vi "CS_Start.vi"() -> ()   [LabVIEW 2014]
doc: "\"Main\" of a CS system on the local machine. Mailny the SuperProc should be started from here. Other objects are created by the SuperProc itself. A list of names of all the objects to be created by the user is part of the data base (SuperProc->Special0-SpecialN).\n\nLicense Agreement for this software:\n\nCopyright (C) 2013 Holger Brand, Dennis Neidherr\nGSI Helmholtzzentrum für Schwerionenforschung GmbH\nPlanckstraße 1\nD-64291 Darmstadt\nGermany\n\nContact: d.neidherr@gsi.de \n\nThis program is free software: you can redistribute it and/or modify it under the terms\nof the GNU General Public License as published by the Free Software Foundation, either\nversion 3 of the License, or (at your option) any later version.\n\nThis program is distributed in the hope that it will be useful, but WITHOUT ANY WARRANTY;\nwithout even the implied warranty of MERCHANTABILITY or FITNESS FOR A PARTICULAR PURPOSE.\nSee the GNU General Public License for more details.\n\nYou should have received a copy of the GNU General Public License along with this program.\nIf not, see <http://www.gnu.org/licenses/>.\n\nFor all questions and ideas contact: d.neidherr@gsi.de or h.brand@gsi.de\nLast update: 20-Mar-2013\n\nmenuHelpStart\nFile\n==\n- \"Shutdown\" gently exits the CS system by removing all objects\n- \"Exit\" unfriendly exits the CS system by exiting the application without removing of objects. \n\nTools\n===\n- \"UserGOG\" displays a generic object GUI (GOG) for on-line testing purposes by the user sitting in front of the computer. If you would like to routinely open a GOG when a CS system starts, please configure a dedicated GOG via the database and configure the SuperProc to create that GOG upon starting up the system.\n\n- \"Inspector\" shows information on the objects of THIS and other CS systems.\n\n- \"DIM Table\" provides a simple possibility for viewing DIM services.\n\n- \"DIM Trend\" can be used for trending of DIM services\n\n- \"DIM Histogram\" can be used for histogramming of multiple DIM services\n\n- \"Access Viewer\" can be used to view the hierarchy of reserved objects. Moreover, it allows for locking the access to certain objects and sub-systems.\n\n- \"DSC Alarm Viewer\" is the alarm viewer of the SCADA backend based on the LabVIEW DSC module. When using the alarm viewer, you will be asked for the name of the DSC interface. The alarm viewer requires a binary compiled with the CSDSC_SCADA package.\nmenuHelpStop\n\ndescriptionHelpStart\n\"Main\" of a CS instance. CS is a framework that can be used by many experiments. CS is a multi-threaded, event driven, object oriented and distributed framework with SCADA functionality. An experiment control system can be developed by combining the CS framework with experiment specific add-ons.\n\nMore information available at http://wiki.gsi.de/cgi-bin/view/CSframework\n\ndescriptionHelpStop"
uses:
  CSClass/CS_Core/GUIs/GOGFrontPanel/GOGFrontPanel.i attribute.ctl
  CSClass/CS_Core/BaseProcess/BaseProcess.descriptor string definition.ctl
  CSClass/CS_Core/CSSystem/CSSystemLib/CSSystemLib.instances options.ctl
  CSlibraries-extern/DimLVEvent/LVDimInterface/LVDimInterface.dim service type.ctl
  CSlibraries/UtilityLib/UtilityLib.helpType.ctl
  CSClass/CS_Core/CSSystem/CoreDefs/CoreDefs.error_severity.ctl
  CSClass/CS_Core/CSSystem/CoreDefs/CoreDefs.error_type.ctl
  CSlibraries/UtilityLib/UtilityLib.valueStatus.ctl
  CSlibraries-extern/DimLVEvent/LVDimInterface/LVDimInterface.dic_info_service_notifier.vi
  CSClass/CS_Core/CSSystem/CoreLib/CoreLib.lvlib
  CSlibraries-extern/DimLVEvent/LVDimInterface/LVDimInterface.lvlib
  CSClass/CS_Core/CSSystem/CSSystemLib/CSSystemLib.lvlib
  CSClass/CS_Core/BaseProcess/BaseProcess.lvlib
  CSlibraries/UtilityLib/UtilityLib.lvlib
  CSClass/CS_Core/CSObj/CSObj.lvlib
  CSClass/CS_Core/CAEObj/CAEObj.lvlib
  CSClass/CS_Core/BaseSM/BaseSM.lvlib
  CSClass/CS_Core/BaseGUI/BaseGUI.lvlib
  CSClass/CS_Core/GUIs/GOGFrontPanel/GOGFrontPanel.lvlib
panel:
  in  "False":bool
  out "database":string="Process@"
  out "domainInfo":string="hello world :-)"
  in  "GOGFrontPanel.i attribute":T1
  out "system running":bool=TRUE
  out "status":string="shutting down..."
  out "systemID":string="TestSystem@KSTest@lxgs11.gsi.de"
  out "error out":errorcluster
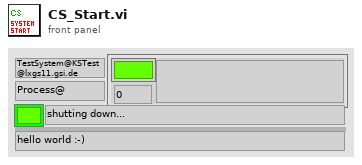
[diagram p1: front panel]
types:
  T1 = typedef "GOGFrontPanel.lvlib/GOGFrontPanel.i attribute.ctl" = cluster{"GOGObject":string, "Object":string, "Method":string, "Descriptor":T2, "Input Descriptor":string, "Output Descriptor":string, "inputNames":string[], "outputNames":string[], "Values":cluster{"descriptor":string, "value":string}[]}
  T2 = typedef "BaseProcess.lvlib/BaseProcess.descriptor string definition.ctl" = string
  T3 = enum32{"Invalid", "Standard", "Closed", "Hidden", "Minimized", "Maximized"}
  T4 = enum32{"invalid app kind", "Development System", "Run Time System", "Student Edition", "Embedded LabVIEW", "Evaluation", "Custom"}
  T5 = typedef "CSSystemLib.lvlib/CSSystemLib.instances options.ctl" = enum16{"add", "delete", "name2ref", "ref2name ", "ref2class", "obj exists?", "cleanup", "get I list", "get I list all", "ref2myclasses", "setClassNames"}
  T6 = enum16{"acquire queue", "release queue", "destroy queue", "get command ID", "destroy all queues"}
  T7 = typedef "UtilityLib.lvlib/UtilityLib.helpType.ctl" = enum16{"unknown", "menu", "description", "about", "special0", "special1", "special2"}
  T8 = typedef "CoreDefs.error_type.ctl" = enum16{"no error", "can't load process", "can't unload process", "process does not exist", "can't install process", "can't remove process", "unknown function", "time out", "can't execute function", "duplicate queue name", "super not found", "caller queue invalid", "can't ping process", "unknown error", "VISA Error", "VISA timeout", "GPIB timeout", "GPIB error", "communication error", "data type mismatch", "can't read data from OPC server", "can't write data to OPC server", "OET error", "function not implemented", "process already exists", "invalid Shared Variable name", "error writing Shared Variable", "error reading Shared Variable", "invalid client name", "corrupt database", "unknown class", "call not authorized", "parameter out of range", "OET timeout: can't get data to modify", "invalid queue name", "requested operation incompatible with current state", "event undefined", "event disabled", "state undefined", "caller is not a friend", "EventBuilder: bad eventID", "EventBuilder: no DAQ devices", "a thread must not stop itself", "UNUSED ELEMENT4", "DiscArchiver: eventData incomplete", "DiscArchiver: eventData does not belong to run", "DiscArchiver: can't open file", "DiscArchiver: can't write to file", "DiscArchiver: available disc space low", "can't acquire semaphore", "error reading data from database", "notifier object is not existing", "can't register process", "can't unregister process", "illegal event type", "object disabled", "object already exists", "can't change state", "Instrument not found", "no connection to remote node", "invalid reference", "N/A", "UNUSED ELEMENT 1", "element not found", "illegal TCP/IP connection detected", "object does not exist", "invalid access ID", "unknown CS system", "invalid privilige", "unsupported data type", "unsupported server type", "IO server already exists", "Shared Variable already exists"}
  T9 = typedef "CoreDefs.error_severity.ctl" = enum16{"undefined", "information", "warning", "error", "fatal"}
  T10 = typedef "UtilityLib.lvlib/UtilityLib.valueStatus.ctl" = enum16{"no info available", "stand by/off", "on", "warning", "alarm/malfunction", "not implemented", "user action required", "important information", "system default", "control default", "indicator default", "button default"}
  T11 = enum32{"Bad", "Idle", "Run top level", "Running"}
  T12 = typedef "LVDimInterface.lvlib/LVDimInterface.dim service type.ctl" = u16
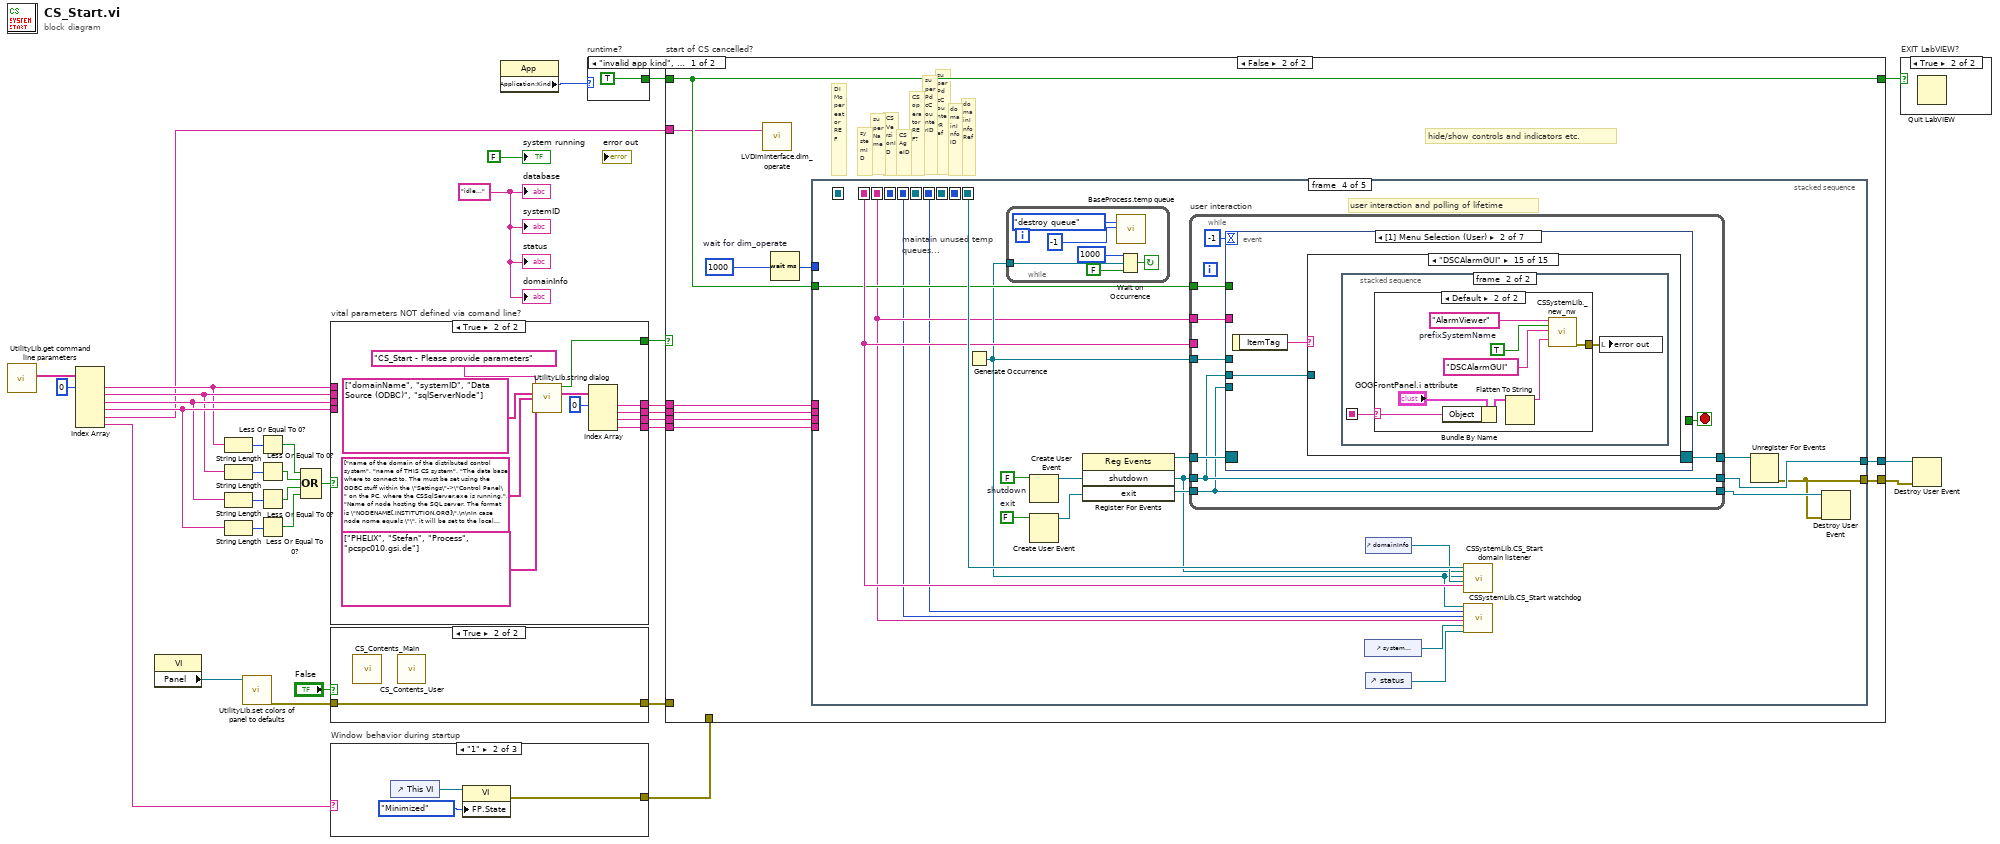
[diagram p0: block diagram]
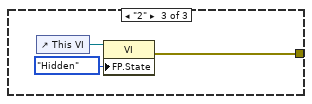
[diagram p3: hidden frame]
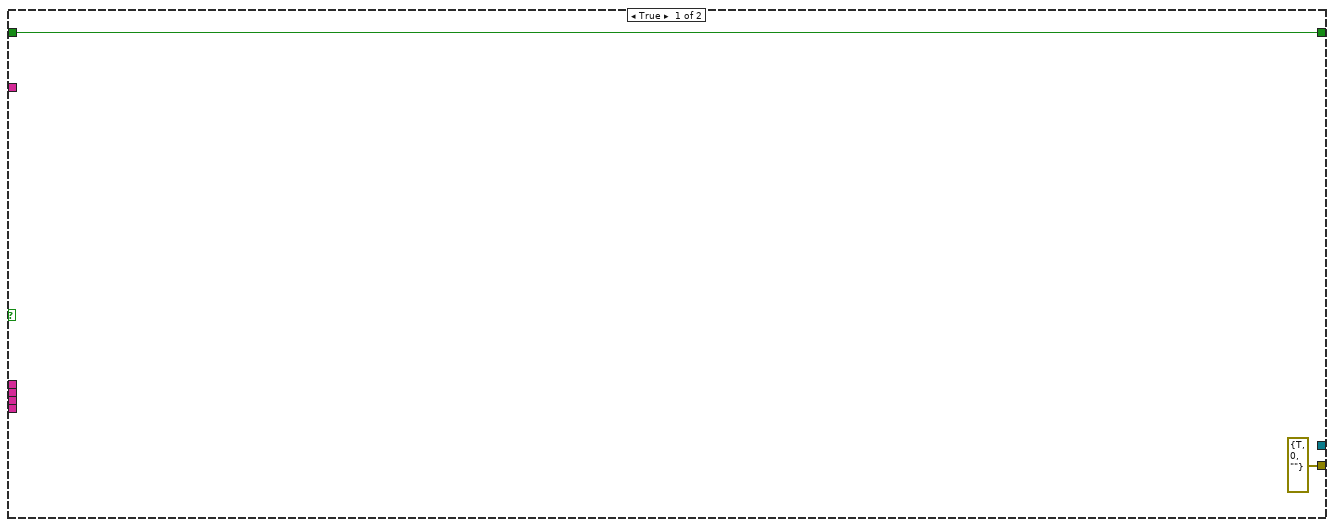
[diagram p6: hidden frame]
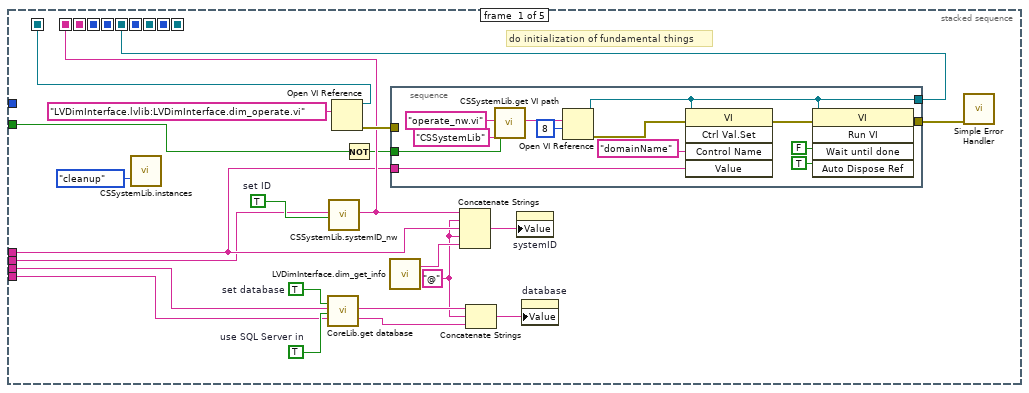
[diagram p7: hidden frame]
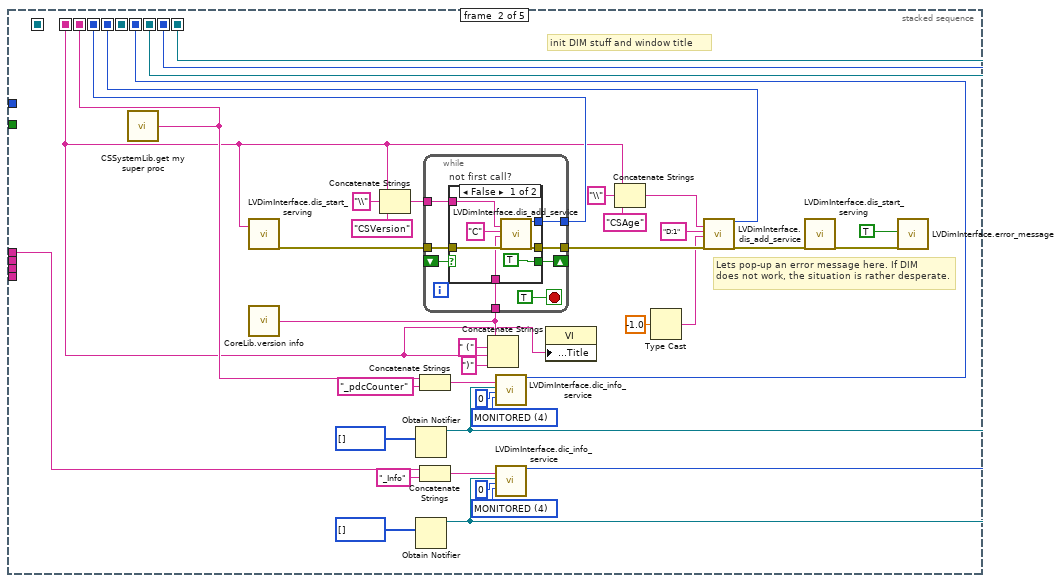
[diagram p8: hidden frame]
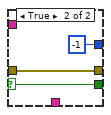
[diagram p9: hidden frame]
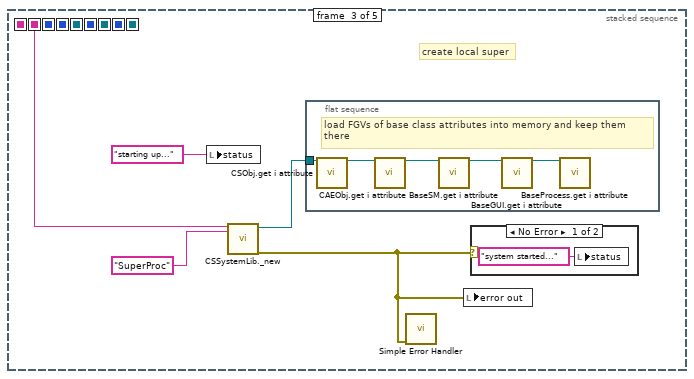
[diagram p10: hidden frame]
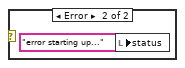
[diagram p11: hidden frame]
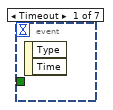
[diagram p12: hidden frame]
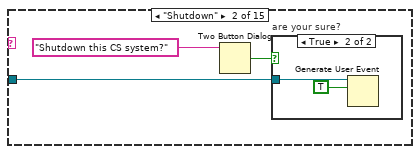
[diagram p14: hidden frame]
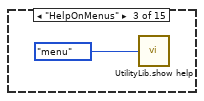
[diagram p16: hidden frame]
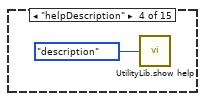
[diagram p17: hidden frame]
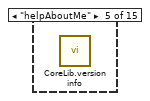
[diagram p18: hidden frame]
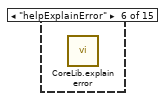
[diagram p19: hidden frame]
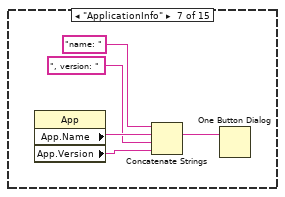
[diagram p20: hidden frame]
diagram:
  w13 = "idle..." ("status")
  n1 = call "UtilityLib.get command line parameters.vi"() -> ("parametersCleaned"=w3:string[])  [unwired: 9 in, 2 out]
  n2 = Index Array(array=w3, index #1=0 ("index")) -> (element #1=w21:string, element #2=w23:string, element #3=w25:string, element #4=w32:string, element #5=w8:string, element #6=w5:string)  [unwired: 5 in]
  n3 = property class="VI"() -> ("Panel"=w9:refnum<vi>)  [unwired: 2 in, 2 out]
  n4 = String Length(string=w21) -> (length=w20:i32)
  n5 = String Length(string=w23) -> (length=w22:i32)
  n6 = String Length(string=w25) -> (length=w24:i32)
  n7 = String Length(string=w32) -> (length=w30:i32)
  n8 = call "UtilityLib.set colors of panel to defaults.vi"("Front Panel"=w9) -> ("error out"=w12:errorcluster)  [unwired: 18 in]
  n9 = Less Or Equal To 0?(x=w20) -> (x <= 0?=w26:bool)
  n10 = Less Or Equal To 0?(x=w22) -> (x <= 0?=w27:bool)
  n11 = Less Or Equal To 0?(x=w24) -> (x <= 0?=w28:bool)
  n12 = Less Or Equal To 0?(x=w30) -> (x <= 0?=w31:bool)
  n13 = Compound Arithmetic op=OR(w26, w27, w28, w31) -> (w29:bool)
  n14 = case "vital parameters NOT defined via comand line?" shown="True" w29 {
    tunnel: [w38 w44] -> w17
    tunnel: w21 -> [w38 _]
    tunnel: [w37 w42] -> w2
    tunnel: w23 -> [w37 _]
    tunnel: w25 -> [w36 _]
    tunnel: [w36 w43] -> w16
    tunnel: w32 -> [w35 _]
    tunnel: [w35 w40] -> w15
    tunnel: [_ w41] -> w6
    frame False {
    }
    frame True {
      n15 = call "UtilityLib.string dialog.vi"("title"="CS_Start - Please provide parameters", "captions"=string[] ["domainName", "systemID", "Data Source (ODBC)", "sqlServerNode"], "helpText"=string[] ["name of the domain of the distributed control system", "name of THIS CS system", "The data base where to connect to. The must be set using the ODBC stuff within the \"Settings\"->\"Control Panel\" on the PC, where the CSSqlServer.exe is running.", "Name of node hosting the SQL server. The format is \"NODENAME[.INSTITUTION.ORG]\".\n\nIn case node nome equals \"\", it will be set to the local host."], "initialValue"=string[] ["PHELIX", "Stefan", "Process", "pcspc010.gsi.de"]) -> ("cancelled"=w41:bool, "strings"=w46:string[])  [unwired: 8 in, 2 out]
      n16 = Index Array(array=w46, index #1=0 ("index")) -> (element #1=w44:string, element #2=w42:string, element #3=w43:string, element #4=w40:string)  [unwired: 3 in]
    }
  }
  n17 = case shown="True" "False" {
    tunnel: w12 -> [w50 w51]
    tunnel: [w50 w51] -> w11
    frame False {
    }
    frame True {
      n18 = call "CS_Contents_Main.vi"() -> ()  [unwired: 1 in]
      n19 = call "CS_Contents_User.vi"() -> ()  [unwired: 1 in]
    }
  }
  n20 = case "Window behavior during startup" shown="\"1\"" w5 {
    tunnel: [_ w54 w55] -> w7
    frame Default {
    }
    frame "1" {
      n21 = control-ref of="This VI"() -> (w52:refnum<vi>)
      n22 = property class="VI"(reference=w52, "FP.State"=T3."Minimized" ("Front Panel Window:State")) -> (error out=w54:errorcluster)  [unwired: 1 in, 1 out]
    }
    frame "2" {
      n23 = control-ref of="This VI"() -> (w57:refnum<vi>)
      n24 = property class="VI"(reference=w57, "FP.State"=T3."Hidden" ("Front Panel Window:State")) -> (error out=w55:errorcluster)  [unwired: 1 in, 1 out]
    }
  }
  n25 = property class="App"() -> ("Application:Kind"=w34:T4)  [unwired: 2 in, 2 out]
  n26 = case "runtime?" shown="\"invalid app kind\", Default" w34 {
    tunnel: [TRUE _] -> w19
    frame "invalid app kind", Default {
    }
    frame "Development System" {
    }
  }
  n27 = case "start of CS cancelled?" shown="False" w6 {
    tunnel: w19 -> [w60 w70]
    tunnel: [w60 w70] -> w18
    tunnel: w8 -> [_ w69]
    tunnel: w17 -> [_ w68]
    tunnel: w2 -> [_ w61]
    tunnel: w16 -> [_ w67]
    tunnel: w15 -> [_ w66]
    tunnel: w11 -> [_ _]
    tunnel: w7 -> [_ _]
    tunnel: [_ w63] -> w4
    tunnel: [errorcluster {"status"=TRUE, "code"=0, "source"=""} ("error out") w62] -> w1
    frame True {
    }
    frame False {
      # "hide/show controls and indicators etc."
      # "domainInfoRef"
      # "domainInfoID"
      # "superPdcCounterRef"
      # "superPdcCounterID"
      # "CSoperator REF?"
      # "CSAgeID"
      # "CSVersionID"
      # "superName"
      # "systemID"
      # "DIMopereator REF"
      n28 = call "LVDimInterface.dim_operate.vi"("DNSNode"=w69) -> ()  [unwired: 19 in]
      n29 = Wait (ms) "wait for dim_operate"(milliseconds to wait=u32 1000) -> (millisecond timer value=w64:u32)
      n30 = stacked-sequence {
        seq-local: [w83 _ _ _ _] -> [_ w106 _ w189 _]
        seq-local: [w90 _ _ _ _] -> [_ _ _ _ w304]
        seq-local: [_ w115 _ _ _] -> [_ _ w162 w182 _]
        seq-local: [_ w130 _ _ _] -> [_ _ _ _ w300]
        seq-local: [_ w129 _ _ _] -> [_ _ _ w178 w299]
        seq-local: [w91 _ _ _ _] -> [_ _ _ _ w303]
        seq-local: [_ w119 _ _ _] -> [_ _ _ w179 w297]
        seq-local: [_ w118 _ _ _] -> [_ _ _ _ w295]
        seq-local: [_ w109 _ _ _] -> [_ _ _ _ w289]
        seq-local: [_ w108 _ _ _] -> [_ _ _ w190 w288]
        tunnel: w70 -> [w73 _ _ w185 w287]
        tunnel: w68 -> [w82 w107 _ _ _]
        tunnel: w61 -> [w71 _ _ _ _]
        tunnel: w67 -> [w86 _ _ _ _]
        tunnel: w66 -> [w85 _ _ _ _]
        tunnel: w64 -> [_ _ _ _ _]
        tunnel: [_ _ _ w177 _] -> w63
        tunnel: [_ _ _ w176 _] -> w62
        frame #0 {
          w80 = "@" ("string")
          w89 = TRUE  # use SQL Server in
          w92 = TRUE  # set database
          w72 = TRUE  # set ID
          # "do initialization of fundamental things"
          n31 = call "CSSystemLib.instances.vi"("Action"=CSSystemLib.instances_options."cleanup") -> ()  [unwired: 12 in, 7 out]
          n32 = call "CoreLib.get database.vi"("set database"=w92, "database in"=w86, "use SQL Server in"=w89, "SQL Server node in"=w85) -> ("database"=w81:string, "SQL Server node"=w79:string)  [unwired: 12 in, 2 out]
          n33 = call "CSSystemLib.systemID_nw.vi"("systemID"=w71, "Force set ID"=w72) -> ("systemID out"=w83:string)  [unwired: 16 in, 1 out]
          n34 = Open VI Reference(vi path="LVDimInterface.lvlib:LVDimInterface.dim_operate.vi") -> (vi reference=w90:refnum<vi>, error out=w87:errorcluster)  [unwired: 5 in]
          n35 = Not(x=w73) -> (.not. x?=w74:bool)
          n36 = call "LVDimInterface.dim_get_info.vi"() -> ("dimDnsNode"=w84:string)  [unwired: 13 in, 6 out]
          n37 = stacked-sequence {
            tunnel: w82 -> [w97]
            tunnel: [w101] -> w91
            tunnel: [w100] -> w75
            tunnel: w87 -> [_]
            tunnel: w74 -> [w94]
            frame #0 {
              n38 = call "CSSystemLib.get VI path.vi"("method"="operate_nw.vi" ("Method"), "class"="CSSystemLib" ("Class"), "reReead"=w94) -> ("VI path"=w96:string)  [unwired: 14 in, 2 out]
              n39 = Open VI Reference(vi path=w96, options=8) -> (vi reference=w101:refnum<vi>, error out=w104:errorcluster)  [unwired: 4 in]
              n40 = invoke class="VI" method="Ctrl Val.Set"(reference=w101, error in=w104, "Control Name"="domainName", "Value"=w97) -> (error out=w103:errorcluster)  [unwired: 1 in, 4 out]
              n41 = invoke class="VI" method="Run VI"(reference=w101, error in=w103, "Wait until done"=FALSE, "Auto Dispose Ref"=TRUE ("Auto Dispose Reference")) -> (error out=w100:errorcluster)  [unwired: 1 in, 4 out]
            }
          }
          n42 = Concatenate Strings(w83, w80, w82, w80, w84) -> (w78:string)
          n43 = Concatenate Strings(w81, w80, w79) -> (w77:string)
          n44 = property on="systemID" class="Str"("Value"=w78) -> ()  [unwired: 2 in, 2 out]
          n45 = property on="database" class="Str"("Value"=w77) -> ()  [unwired: 2 in, 2 out]
          n46 = call <vilib>:"Simple Error Handler.vi"("error in (no error)"=w75) -> ()  [unwired: 4 in, 5 out]
        }
        frame #1 {
          w114 = T12 4 items=["ONCE_ONLY"=1, "TIMED"=2, "MONITORED"=4] ("serviceType")
          w116 = T12 4 items=["ONCE_ONLY"=1, "TIMED"=2, "MONITORED"=4] ("serviceType")
          # "Lets pop-up an error message here. If DIM\ndoes not work, the situation is rather desperate."
          # "init DIM stuff and window title"
          n47 = call "CSSystemLib.get my super proc.vi"() -> ("name"=w115:string)  [unwired: 1 in]
          n48 = call "LVDimInterface.dis_start_serving.vi"("serverName"=w106) -> ("error out"=w138:errorcluster)  [unwired: 17 in, 1 out]
          n49 = call "CoreLib.version info.vi"() -> ("CS Version"=w126:string)  [unwired: 4 in, 1 out]
          n50 = Concatenate Strings(w106, "\\" ("string"), "CSVersion" ("string")) -> (w141:string)
          n51 = Obtain Notifier(notification data type=i8[] []) -> (notifier out=w118:refnum<notifier>)  [unwired: 3 in, 2 out]
          n52 = Obtain Notifier(notification data type=i8[] []) -> (notifier out=w108:refnum<notifier>)  [unwired: 3 in, 2 out]
          n53 = Concatenate Strings(w115, "_pdcCounter" ("string")) -> (w121:string)
          n54 = Concatenate Strings(w107, "_Info" ("string")) -> (w111:string)
          n55 = while {
            tunnel: w141 -> [w149]
            tunnel: w138 -> [w148]
            tunnel: [w147] -> w134
            tunnel: [w146] -> w130
            tunnel: w126 -> [w145]
            shift-right: [w143] -> _
            shift-left: _ -> [w142]
            stop <- TRUE stop-if-true
            n56 = case "not first call?" shown="False" w142 {
              selector: w142 -> [_ w157]
              tunnel: w149 -> [w156 _]
              tunnel: w148 -> [w154 w159]
              tunnel: [w153 w159] -> w147
              tunnel: [w152 -1 ("my_serviceID")] -> w146
              tunnel: w145 -> [w151 _]
              tunnel: [TRUE w157] -> w143
              frame False {
                n57 = call "LVDimInterface.dis_add_service.vi"("serviceName"=w156, "typeDescriptor"="C", "data"=w151, "error in (no error)"=w154) -> ("my_serviceID"=w152:i32, "error out"=w153:errorcluster)  [unwired: 14 in]
              }
              frame True {
              }
            }
          }
          n58 = Concatenate Strings(w126, " (" ("string"), w106, ")" ("string")) -> ()  [unwired: 1 out]
          n59 = call-poly "LVDimInterface.dic_info_service.vi"("serviceName"=w121, "notifierRef"=w118, "timeout [s]"=0, "serviceType"=w116) -> ("callBackID"=w119:i32)  [unwired: 14 in, 1 out]
          n60 = call-poly "LVDimInterface.dic_info_service.vi"("serviceName"=w111, "notifierRef"=w108, "timeout [s]"=0, "serviceType"=w114) -> ("callBackID"=w109:i32)  [unwired: 14 in, 1 out]
          n61 = property class="VI"("Front Panel Window:Title"=w106) -> ()  [unwired: 2 in, 2 out]
          n62 = Concatenate Strings(w106, "\\" ("string"), "CSAge" ("string")) -> (w137:string)
          n63 = Type Cast(x=-1.0) -> (*(type *) &x=w132:string)  [unwired: 1 in]
          n64 = call "LVDimInterface.dis_add_service.vi"("serviceName"=w137, "typeDescriptor"="D:1", "data"=w132, "error in (no error)"=w134) -> ("my_serviceID"=w129:i32, "error out"=w124:errorcluster)  [unwired: 14 in]
          n65 = call "LVDimInterface.dis_start_serving.vi"("error in (no error)"=w124) -> ("error out"=w123:errorcluster)  [unwired: 17 in, 1 out]
          n66 = call "LVDimInterface.error_message.vi"("add message to source"=TRUE, "error in (no error)"=w123) -> ()  [unwired: 14 in, 4 out]
        }
        frame #2 {
          # "create local super"
          n67 = local write "status"("starting up..." ("status")) -> ()
          n68 = call "CSSystemLib._new.vi"("object name"=w162, "class name"="SuperProc") -> ("i ref out"=w161:refnum<vi>, "error out"=w160:errorcluster)  [unwired: 14 in, 2 out]
          n69 = flat-sequence {
            tunnel: w161 -> [w169]
            frame #0 {
              # "load FGVs of base class attributes into memory and keep them\nthere"
              n70 = call "CSObj.get i attribute.vi"("i ref in"=w169) -> ("i ref out"=w168:refnum<vi>)  [unwired: 16 in, 2 out]
              n71 = call "CAEObj.get i attribute.vi"("i ref in"=w168) -> ("i ref out"=w167:refnum<vi>)  [unwired: 16 in, 2 out]
              n72 = call "BaseSM.get i attribute.vi"("i ref in"=w167) -> ("i ref out"=w166:refnum<vi>)  [unwired: 16 in, 2 out]
              n73 = call "BaseGUI.get i attribute.vi"("i ref in"=w166) -> ("i ref out"=w165:refnum<vi>)  [unwired: 16 in, 2 out]
              n74 = call "BaseProcess.get i attribute.vi"("i ref in"=w165) -> ()  [unwired: 16 in, 3 out]
            }
          }
          n75 = call <vilib>:"Simple Error Handler.vi"("error in (no error)"=w160) -> ()  [unwired: 4 in, 5 out]
          n76 = local write "error out"(w160) -> ()
          n77 = case shown="No Error" w160 {
            frame No Error {
              n78 = local write "status"("system started..." ("status")) -> ()
            }
            frame Error {
              n79 = local write "status"("error starting up..." ("status")) -> ()
            }
          }
        }
        frame #3 {
          w174 = FALSE  # exit
          w175 = FALSE  # shutdown
          # "user interaction and polling of lifetime"
          n80 = Generate Occurrence() -> (w183:refnum<k4>)
          n81 = while "maintain unused temp queues..." {
            tunnel: w183 -> [w194]
            stop <- w195 continue-if-true
            n82 = Wait on Occurrence(1:FALSE ("ignore previous (T)"), 2:w194, 3:1000 ("ms timeout (-1)")) -> (0:w195:bool)
            n83 = call "BaseProcess.temp queue.vi"("Action"=T6."destroy queue", "ID in"=-1) -> ()  [unwired: 14 in, 4 out]
          }
          n84 = Create User Event(user event datatype=w175) -> (user event=w172:refnum<user-event>)  [unwired: 1 in, 1 out]
          n85 = Create User Event(user event datatype=w174) -> (user event=w173:refnum<user-event>)  [unwired: 1 in, 1 out]
          n86 = register-events(w172, w173) -> (reference out=w188:refnum<event-registration>)  [unwired: 2 in, 1 out]
          n87 = while "user interaction" {
            tunnel: w183 -> [w205]
            tunnel: w182 -> [w203]
            tunnel: w189 -> [_]
            tunnel: w185 -> [w201]
            tunnel: w188 -> [w200]
            tunnel: w172 -> [w199]
            tunnel: [w198] -> w187
            tunnel: [w199] -> w177
            tunnel: w173 -> [w197]
            tunnel: [w197] -> w186
            stop <- w204 stop-if-true
            n88 = event shown="[1] Menu Selection (User)" {
              selector: w200 -> [_ _ _ _ _ _ _]
              dyn-events: [_ _ _ _ _ _ _] -> w198
              timeout: -1 -> [_ _ _ _ _ _ _]
              tunnel: w205 -> [_ _ _ w270 _ _ _]
              tunnel: w203 -> [_ _ _ w269 _ _ _]
              tunnel: [_ _ _ w268 _ _ _] -> w204
              tunnel: w201 -> [_ _ _ _ _ _ w282]
              tunnel: w199 -> [_ w206 _ _ _ _ _]
              tunnel: w197 -> [_ _ _ _ w277 w281 _]
              event Timeout {
                n89 = event-data() -> ()  [unwired: 1 in, 2 out]
              }
              event Menu Selection (User) {
                n90 = event-data() -> ("ItemTag"=w207:string)  [unwired: 1 in]
                n91 = case shown="\"DSCAlarmGUI\"" w207 {
                  tunnel: w206 -> [_ w208 _ _ _ _ _ _ _ _ _ _ _ _ _]
                  frame Default {
                  }
                  frame "Shutdown" {
                    n92 = Two Button Dialog(message="Shutdown this CS system?") -> (T button?=w209:bool)  [unwired: 2 in]
                    n93 = case "are your sure?" shown="True" w209 {
                      tunnel: w208 -> [_ w211]
                      frame False {
                      }
                      frame True {
                        n94 = Generate User Event(user event=w211, event data cluster=TRUE ("event data")) -> ()  [unwired: 2 in, 2 out]
                      }
                    }
                  }
                  frame "HelpOnMenus" {
                    n95 = call "UtilityLib.show help.vi"("helpType"=UtilityLib.helpType."menu") -> ()
                  }
                  frame "helpDescription" {
                    n96 = call "UtilityLib.show help.vi"("helpType"=UtilityLib.helpType."description") -> ()
                  }
                  frame "helpAboutMe" {
                    n97 = call "CoreLib.version info.vi"() -> ()  [unwired: 4 in, 2 out]
                  }
                  frame "helpExplainError" {
                    n98 = call "CoreLib.explain error.vi"() -> ()  [unwired: 1 in]
                  }
                  frame "ApplicationInfo" {
                    n99 = property class="App"() -> ("App.Name"=w217:string, "App.Version"=w215:string)  [unwired: 2 in, 2 out]
                    n100 = Concatenate Strings("name: " ("string"), w217, ", version: " ("string"), w215) -> (w219:string)
                    n101 = One Button Dialog(message=w219) -> ()  [unwired: 1 in, 1 out]
                  }
                  frame "UserGOG" {
                    w223 = TRUE  # prefixSystemName
                    n102 = call "CSSystemLib._new_nw.vi"("objectName"="UserGOG", "prefixSystemName"=w223, "className"="GeneralObjectGUI", "data in"="N/A") -> ("error out"=w222:errorcluster)  [unwired: 13 in, 2 out]
                    n103 = local write "error out"(w222) -> ()
                  }
                  frame "Inspector" {
                    w228 = TRUE  # prefixSystemName
                    n104 = call "CSSystemLib._new_nw.vi"("objectName"="Inspector" ("Data"), "prefixSystemName"=w228, "className"="ObjectInspector", "data in"="N/A") -> ("error out"=w227:errorcluster)  [unwired: 13 in, 2 out]
                    n105 = local write "error out"(w227) -> ()
                  }
                  frame "DIMTable" {
                    w233 = TRUE  # prefixSystemName
                    n106 = call "CSSystemLib._new_nw.vi"("objectName"="DIMTable" ("Data"), "prefixSystemName"=w233, "className"="DIMTableView", "data in"="N/A") -> ("error out"=w232:errorcluster)  [unwired: 13 in, 2 out]
                    n107 = local write "error out"(w232) -> ()
                  }
                  frame "DIMTrendGUI" {
                    w238 = TRUE  # prefixSystemName
                    n108 = call "CSSystemLib._new_nw.vi"("objectName"="DIMTrend" ("Data"), "prefixSystemName"=w238, "className"="DIMTrendGUI", "data in"="N/A") -> ("error out"=w237:errorcluster)  [unwired: 13 in, 2 out]
                    n109 = local write "error out"(w237) -> ()
                  }
                  frame "DIMHistogramGUI" {
                    w243 = TRUE  # prefixSystemName
                    n110 = call "CSSystemLib._new_nw.vi"("objectName"="DIMHistogram" ("Data"), "prefixSystemName"=w243, "className"="DIMHistogramGUI", "data in"="N/A") -> ("error out"=w242:errorcluster)  [unwired: 13 in, 2 out]
                    n111 = local write "error out"(w242) -> ()
                  }
                  frame "ToolsDispatchMessageBox" {
                    n112 = call "CSSystemLib.CS_Start dispatch message box.vi"() -> ("error out"=w245:errorcluster)  [unwired: 18 in, 1 out]
                    n113 = local write "error out"(w245) -> ()
                  }
                  frame "AccessViewer" {
                    w249 = TRUE  # prefixSystemName
                    n114 = call "CSSystemLib._new_nw.vi"("objectName"="AccessViewer" ("Data"), "prefixSystemName"=w249, "className"="CSAccessViewer", "data in"="N/A") -> ("error out"=w248:errorcluster)  [unwired: 13 in, 2 out]
                    n115 = local write "error out"(w248) -> ()
                  }
                  frame "DSCAlarmGUI" {
                    n116 = stacked-sequence {
                      seq-local: [w251 _] -> [_ w253]
                      frame #0 {
                        n117 = call "CSSystemLib._getInstances_nw.vi"() -> ("i list"=w252:string[])  [unwired: 18 in, 1 out]
                        n118 = call "UtilityLib.selectName.vi"("names"=w252) -> ("name"=w251:string)  [unwired: 16 in, 2 out]
                      }
                      frame #1 {
                        n119 = case shown="Default" w253 {
                          selector: w253 -> [_ w258]
                          tunnel: [w257 w263] -> w254
                          frame "" {
                            n120 = call "CoreLib.my to LV error.vi"("ErrorTypes"=CoreDefs.error_type."process does not exist", "severityLevel"=CoreDefs.error_severity."information") -> ("myErrorCluster"=w257:errorcluster)  [unwired: 16 in, 1 out]
                          }
                          frame Default {
                            w264 = TRUE  # prefixSystemName
                            n121 = Bundle By Name(cluster="GOGFrontPanel.i attribute", "Object"=w258) -> (w260:T1)
                            n122 = Flatten To String(anything=w260) -> (data string=w259:string)  [unwired: 3 in, 2 out]
                            n123 = call "CSSystemLib._new_nw.vi"("objectName"="AlarmViewer" ("Data"), "prefixSystemName"=w264, "className"="DSCAlarmGUI", "data in"=w259) -> ("error out"=w263:errorcluster)  [unwired: 13 in, 2 out]
                          }
                        }
                        n124 = local write "error out"(w254) -> ()
                      }
                    }
                  }
                }
              }
              event "domainInfo": Mouse Down {
                n125 = event-data() -> ()  [unwired: 1 in, 1 out]
                n126 = control-ref of="domainInfo"() -> (w267:refnum<vi>)
                n127 = call "UtilityLib.set color of simple string or numeric.vi"("simpleString"=w267, "valueStatus"=UtilityLib.valueStatus."indicator default") -> ()  [unwired: 17 in, 1 out]
              }
              event User Event {
                n128 = event-data() -> ("shutdown"=w268:bool)  [unwired: 1 in]
                n129 = case "shutdown?" shown="True" w268 {
                  tunnel: w269 -> [_ w275]
                  tunnel: w270 -> [_ w273]
                  frame False {
                  }
                  frame True {
                    n130 = Set Occurrence(w273) -> ()
                    n131 = call "CSSystemLib.name2ref.vi"("name"=w275) -> ("obj refnum"=w272:refnum<vi>)
                    n132 = call "CSSystemLib._delete.vi"("i ref"=w272) -> ("error out"=w271:errorcluster)  [unwired: 18 in]
                    n133 = property on="error out" class="Clust (strict)"("Value"=w271) -> ()  [unwired: 2 in, 2 out]
                    n134 = local write "status"("shutting down..." ("status")) -> ()
                  }
                }
              }
              event Panel Close? {
                n135 = event-data() -> ()  [unwired: 1 in, 1 out]
                n136 = Generate User Event(user event=w277, event data cluster=TRUE ("event data")) -> ()  [unwired: 2 in, 2 out]
                n137 = event-data("Discard?"=TRUE) -> ()  [unwired: 1 in, 1 out]
              }
              event Application Instance Close? {
                n138 = event-data() -> ()  [unwired: 1 in, 1 out]
                n139 = Generate User Event(user event=w281, event data cluster=TRUE ("event data")) -> ()  [unwired: 2 in, 2 out]
                n140 = event-data("Discard?"=TRUE) -> ()  [unwired: 1 in, 1 out]
              }
              event User Event {
                n141 = event-data() -> ()  [unwired: 1 in, 1 out]
                n142 = Two Button Dialog(message="Exit this CS system without shutdown?") -> (T button?=w283:bool)  [unwired: 2 in]
                n143 = case "exit CS?" shown="False" w282 {
                  tunnel: w283 -> [_ w286]
                  frame False {
                    n144 = One Button Dialog(message="\"EXIT\" is not available in the development system. ") -> ()  [unwired: 1 in, 1 out]
                  }
                  frame True {
                    n145 = case "Exit application?" shown="True" w286 {
                      frame False {
                      }
                      frame True {
                        n146 = Quit LabVIEW() -> ()  [unwired: 1 in]
                      }
                    }
                  }
                }
              }
            }
          }
          n147 = control-ref of="system running"() -> (w181:refnum<vi>)
          n148 = control-ref of="domainInfo"() -> (w184:refnum<vi>)
          n149 = control-ref of="status"() -> (w180:refnum<vi>)
          n150 = call "CSSystemLib.CS_Start domain listener.vi"("domainInfo"=w190, "shutdown"=w172, "stop"=w183, "domainInfoDisplay"=w184, "systemID"=w189) -> ()  [unwired: 15 in]
          n151 = call "CSSystemLib.CS_Start watchdog.vi"("stop"=w183, "superPdcCounterID"=w179, "CSAgeID"=w178, "superName"=w182, "systemRunning"=w181, "status"=w180) -> ()  [unwired: 14 in]
          n152 = Unregister For Events(event registration refnum=w187) -> (error out=w176:errorcluster)  [unwired: 1 in]
          n153 = Destroy User Event(user event=w186, error in=w176) -> ()  [unwired: 1 out]
        }
        frame #4 {
          # "shut down DIM stuff"
          n154 = flat-sequence {
            tunnel: [w310] -> w294
            frame #0 {
              n155 = call "BaseProcess.temp queue.vi"("Action"=T6."destroy all queues") -> ()  [unwired: 15 in, 4 out]
              n156 = call "CSSystemLib.updateInstanceList_nw.vi"("remove list"=TRUE) -> ()  [unwired: 4 in]
            }
            frame #1 {
              n157 = call "LVDimInterface.dis_start_serving.vi"("serverName"="dummy") -> ("error out"=w310:errorcluster)  [unwired: 17 in, 1 out]
            }
          }
          n158 = call "LVDimInterface.dic_release_service.vi"("callBackID"=w289) -> ("error out"=w291:errorcluster)  [unwired: 18 in]
          n159 = call "LVDimInterface.dic_release_service.vi"("callBackID"=w297) -> ("error out"=w296:errorcluster)  [unwired: 18 in]
          n160 = case shown="False" FALSE ("Case Constant\n(See Context Help)") {
            tunnel: [_ w306] -> w301
            tunnel: w300 -> [_ w305]
            frame False {
            }
            frame True {
              # "always keep\none service!"
              n161 = call "LVDimInterface.dis_remove_service.vi"("my_serviceID"=w305) -> ("error out"=w306:errorcluster)  [unwired: 18 in]
            }
          }
          n162 = Release Notifier(notifier=w288, error in (no error)=w291) -> (error out=w290:errorcluster)  [unwired: 1 in, 2 out]
          n163 = Release Notifier(notifier=w295, error in (no error)=w296) -> (error out=w292:errorcluster)  [unwired: 1 in, 2 out]
          n164 = call "LVDimInterface.dis_remove_service.vi"("my_serviceID"=w299, "error in (no error)"=w301) -> ("error out"=w298:errorcluster)  [unwired: 17 in]
          n165 = case "runtime system?" shown="False" w287 {
            tunnel: w304 -> [w315 w328]
            tunnel: w303 -> [w312 w329]
            tunnel: [w312 w329] -> w302
            tunnel: w298 -> [_ _]
            tunnel: w294 -> [_ _]
            tunnel: w292 -> [_ _]
            tunnel: w290 -> [_ _]
            frame False {
              n166 = flat-sequence {
                tunnel: w315 -> [w317]
                tunnel: [w317] -> w314
                tunnel: w312 -> [w316]
                tunnel: w314 -> [w324]
                frame #0 {
                  n167 = while {
                    tunnel: w316 -> [w322]
                    stop <- w320 stop-if-true
                    n168 = property class="VI"(reference=w322) -> ("Execution:State"=w321:T11)  [unwired: 1 in, 2 out]
                    n169 = Less Or Equal?(x=w321, y=T11."Idle" ("Execution:State")) -> (x <= y?=w320:bool)
                    n170 = Wait Until Next ms Multiple(millisecond multiple=u32 250) -> ()  [unwired: 1 out]
                  }
                }
                frame #1 {
                  n171 = invoke class="VI" method="Ctrl Val.Set"(reference=w324, "Control Name"="stop", "Value"=TRUE) -> (error out=w325:errorcluster)  [unwired: 2 in, 4 out]
                  n172 = Close Reference(reference=w324, error in (no error)=w325) -> ()  [unwired: 1 out]
                }
              }
              n173 = invoke class="VI" method="Ctrl Val.Set"(reference=w312, "Control Name"="stop", "Value"=TRUE) -> ()  [unwired: 2 in, 5 out]
            }
            frame True {
              n174 = flat-sequence {
                tunnel: w328 -> [w330]
                tunnel: [w330] -> w327
                tunnel: w327 -> [w331]
                frame #0 {
                  n175 = call "LVDimInterface.dis_stop_serving.vi"() -> ()  [unwired: 19 in, 1 out]
                }
                frame #1 {
                  n176 = invoke class="VI" method="Ctrl Val.Set"(reference=w331, "Control Name"="stop", "Value"=TRUE) -> ()  [unwired: 2 in, 5 out]
                }
              }
            }
          }
          n177 = Close Reference(reference=w302) -> ()  [unwired: 1 in, 1 out]
        }
      }
    }
  }
  n178 = case "EXIT LabVIEW?" shown="True" w18 {
    frame False {
    }
    frame True {
      n179 = Quit LabVIEW() -> ()  [unwired: 1 in]
    }
  }
  n180 = Destroy User Event(user event=w4, error in=w1) -> ()  [unwired: 1 out]
  "status" <- w13
  "domainInfo" <- w13
  "system running" <- FALSE ("system running")
  "systemID" <- w13
  "database" <- w13
